vi "determineConfigurationDirectoryPathWindows.vi"(8 "error in (no error)":errorcluster, 11 "Target in":refnum<class "Target.lvclass">) -> (0 "error out":errorcluster, 2 "configDirectoryPathWindows":path, 3 "Target out":refnum<class "Target.lvclass">)   [LabVIEW 2012, in "Target.lvclass"]
doc: "Returns the configuration directory path applicable on a Windows target. The method on the abstract class returns an empty path."
uses:
  Target.lvclass
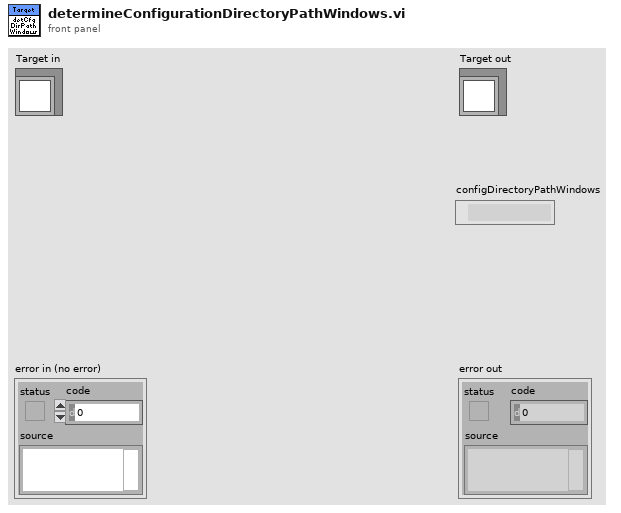
[diagram p1: front panel]
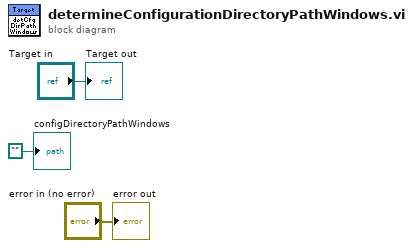
[diagram p0: block diagram]
diagram:
  "error out" <- "error in (no error)"
  "Target out" <- "Target in"
  "configDirectoryPathWindows" <- path ""
